vi "Setup.vi"(10 "Actor":refnum<class "Actor.lvclass">, 11 "Dev Actor in":refnum<class "Dev Actor.lvclass">) -> (3 "Dev Actor out":refnum<class "Dev Actor.lvclass">)   [LabVIEW 2021, in "Dev Actor.lvlib" / "Dev Actor.lvclass"]
uses:
  Dev Actor.lvclass
  Dev Actor.lvclass/Dev Actor.ctl
  Dev Panel/Dev Panel.lvclass
  src/Actor/Actor/Actor.lvclass
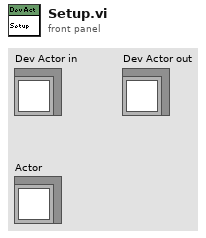
[diagram p1: front panel]
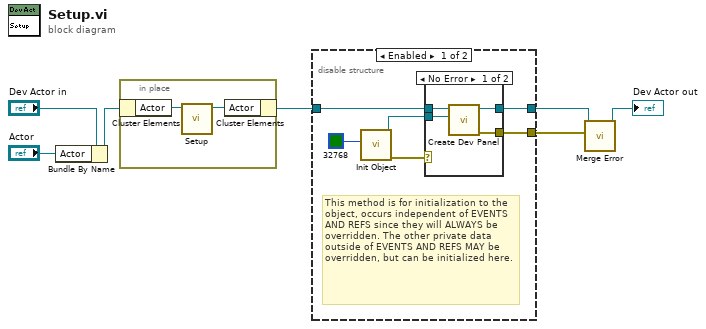
[diagram p0: block diagram]
diagram:
  n1 = Bundle By Name(cluster="Dev Actor in", "Actor"="Actor") -> (w6:refnum<class "Dev Actor.lvclass">)
  n2 = in-place {
    n3 = in-place-cluster #1(w6) -> ("Actor"=w8:refnum<class "Actor.lvclass">)
    n4 = call-dynamic "Setup.vi"("Actor in"=w8) -> ("Actor out"=w9:refnum<class "Actor.lvclass">)  [unwired: 10 in]
    n5 = in-place-cluster #1("Actor"=w9) -> (w2:refnum<class "Dev Actor.lvclass">)
  }
  n6 = disable-structure shown="Enabled" {
    disable-tunnel: [w15 _] -> w3
    disable-tunnel: w2 -> [w14 _]
    disable-tunnel: [w13 _] -> w1
    frame Enabled {
      # "This method is for initialization to the object, occurs independent of EVENTS AND REFS since they will ALWAYS be overridden. The other private data outside of EVENTS AND REFS MAY be overridden, but can be initialized here."
      n7 = call "Init Object.vi"("BG Color"=u32 32768) -> ("error out"=w11:errorcluster, "Dev Panel out"=w12:refnum<class "Dev Panel.lvclass">)  [unwired: 9 in]
      n8 = case shown="No Error" w11 {
        selector: w11 -> [_ w20]
        tunnel: [w19 w20] -> w15
        tunnel: w14 -> [w18 w21]
        tunnel: [w17 w21] -> w13
        tunnel: w12 -> [w16 _]
        frame No Error {
          n9 = call "Create Dev Panel.vi"("Dev Panel"=w16, "Dev Actor in"=w18) -> ("error out"=w19:errorcluster, "Dev Actor out"=w17:refnum<class "Dev Actor.lvclass">)  [unwired: 8 in]
        }
        frame Error {
        }
      }
    }
    frame Disabled {
    }
  }
  n10 = call-dynamic "Merge Error.vi"("Error"=w3, "Dev Actor in"=w1) -> ("Dev Actor out"=→"Dev Actor out":refnum<class "Dev Actor.lvclass">)  [unwired: 9 in]
